vi "Image Processing.vi"(0 "File Path":path, 1 "Lithography Information":T2(array[cluster]), 2 "Crop?":bool, 3 "Crop Data":T3, 4 "Angle (degrees)":dbl, 5 "error in (no error)":errorcluster, 6 "Size":cluster{"Width":dbl, "Height":dbl}, 7 "Page":i32) -> (14 "Image Out":T4(plugin-control), 15 "Offset":T1, 16 "Sample Size":cluster{"Width (µm)":dbl, "Height (µm)":dbl}, 19 "error out":errorcluster)   [LabVIEW 2011]
uses:
  <vilib>/vision/NI_Vision_Development_Module.lvlib
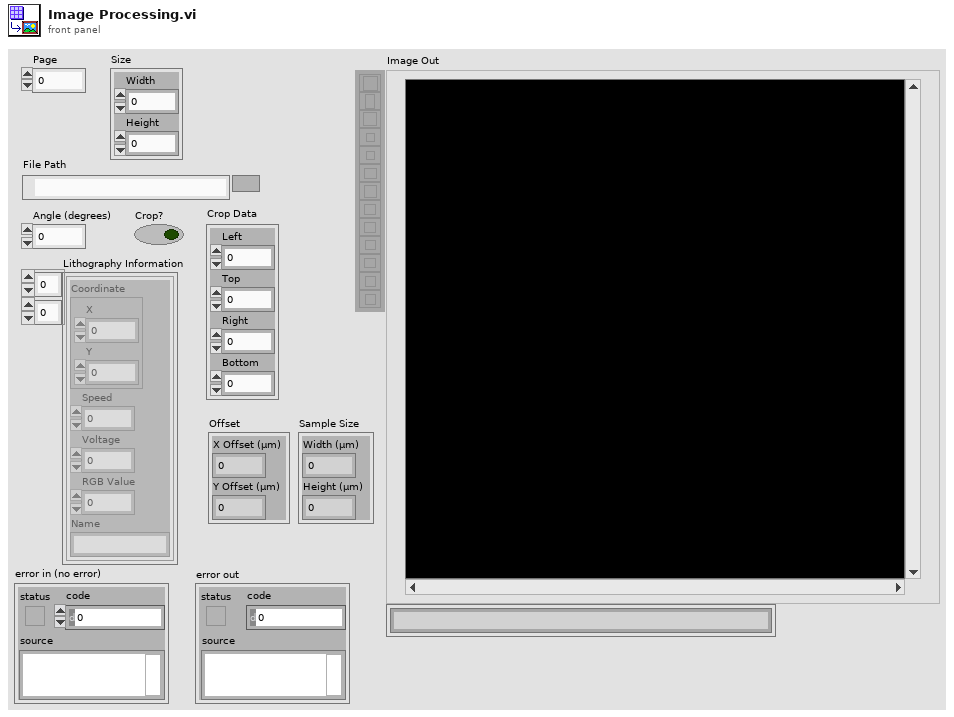
[diagram p1: front panel]
types:
  T1 = cluster{"X Offset (µm)":dbl, "Y Offset (µm)":dbl}
  T2 = cluster{"Coordinate":cluster{"X":dbl, "Y":dbl}, "Speed":dbl, "Voltage":dbl, "RGB Value":i32, "Name":string}[][]
  T3 = cluster{"Left":dbl, "Top":dbl, "Right":dbl, "Bottom":dbl}
  T4 = typedef "IMAQ Image.ctl" = refnum<image>
  T5 = typedef "Image Type" = u32
  T6 = cluster{"Coordinate":cluster{"X":dbl, "Y":dbl}, "Speed":dbl, "Voltage":dbl, "RGB Value":i32, "Name":string}
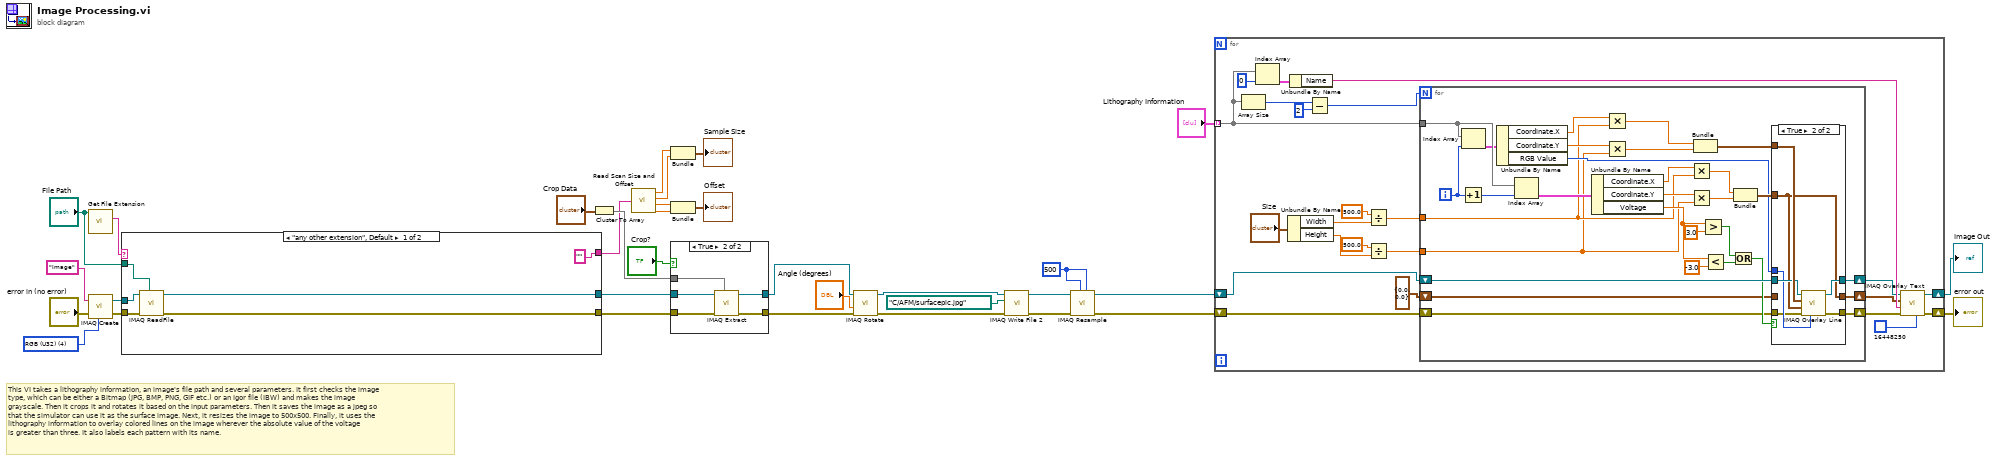
[diagram p0: block diagram]
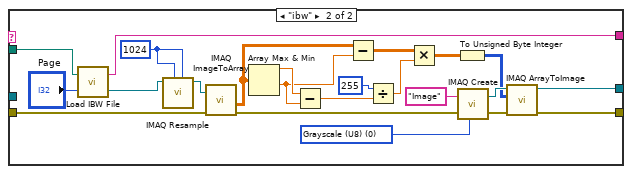
[diagram p2: hidden frame]
diagram:
  w10 = 500 ("Y Resolution")
  w32 = T5 4 items=["Grayscale (U8)", "Grayscale (I16)", "Grayscale (SGL)", "Complex (CSG)", "RGB (U32)", "HSL (U32)", "RGB (U64)", "Grayscale (U16)"] ("Image Type")
  # "This VI takes a lithography information, an image's file path and several parameters. It first checks the image \ntype, which can be either a Bitmap (JPG, BMP, PNG, GIF etc.) or an Igor file (IBW) and makes the image \ngrayscale. Then it crops it and rotates it based on the input parameters. Then it saves the image as a jpeg so \nthat the simulator can use it as the surface image. Next, it resizes the image to 500x500. Finally, it uses the \nlithography information to overlay colored lines on the image wherever the absolute value of the voltage \nis greater than three. It also labels each pattern with its name."
  n1 = call <vilib>:"Get File Extension.vi"("file"="File Path") -> ("lowercase file extension"=w19:string)  [unwired: 7 in, 3 out]
  n2 = call "IMAQ Create"("Image Name"="Image", "Image Type"=w32, "error in (no error)"="error in (no error)") -> ("New Image"=w31:T4, "error out"=w30:errorcluster)  [unwired: 2 in]
  n3 = case shown="\"any other extension\", Default" w19 {
    tunnel: w31 -> [w39 _]
    tunnel: w30 -> [w38 w60]
    tunnel: [w37 w53] -> w29
    tunnel: [w36 w52] -> w28
    tunnel: "File Path" -> [w35 w62]
    tunnel: ["" ("Wave Note") w40] -> w7
    frame "any other extension", Default {
      n4 = call "IMAQ ReadFile"("File Path"=w35, "error in (no error)"=w38, "Image"=w39) -> ("error out"=w36:errorcluster, "Image Out"=w37:T4)  [unwired: 4 in, 3 out]
    }
    frame "ibw" {
      w50 = 1024 ("Y Resolution")
      w57 = T5 0 items=["Grayscale (U8)", "Grayscale (I16)", "Grayscale (SGL)", "Complex (CSG)", "RGB (U32)", "HSL (U32)", "RGB (U64)", "Grayscale (U16)"] ("Image Type")
      n5 = call "Load IBW File.vi"("Page"="Page", "file path (dialog if empty)"=w62) -> ("Image"=w49:T4, "Wave Note"=w40:string)
      n6 = call "IMAQ Resample"("X Resolution"=w50, "Y Resolution"=w50, "Image Src"=w49) -> ("Image Dst Out"=w48:T4)  [unwired: 7 in, 1 out]
      n7 = call "IMAQ ImageToArray"("error in (no error)"=w60, "Image"=w48) -> ("Image Pixels (Float)"=w59:sgl[][], "error out"=w54:errorcluster)  [unwired: 2 in, 3 out]
      n8 = Array Max & Min(array=w59) -> (max value=w47:sgl, min value=w46:sgl)  [unwired: 2 out]
      n9 = Subtract(x=w47, y=w46) -> (x-y=w44:sgl)
      n10 = Subtract(x=w59, y=w46) -> (x-y=w45:sgl[][])
      n11 = Divide(x=255, y=w44) -> (x/y=w42:sgl)
      n12 = Multiply(x=w45, y=w42) -> (x*y=w41:sgl[][])
      n13 = To Unsigned Byte Integer(number=w41) -> (unsigned 8bit integer=w56:u8[][])
      n14 = call "IMAQ Create"("Image Name"="Image", "Image Type"=w57, "error in (no error)"=w54) -> ("New Image"=w58:T4, "error out"=w55:errorcluster)  [unwired: 2 in]
      n15 = call "IMAQ ArrayToImage"("error in (no error)"=w55, "Image Pixels (U8)"=w56, "Image"=w58) -> ("error out"=w52:errorcluster, "Image Out"=w53:T4)  [unwired: 7 in]
    }
  }
  n16 = Cluster To Array(cluster="Crop Data") -> (array=w26:dbl[])
  n17 = call "Read Scan Size and Offset.vi"("Read in the string file"=w7) -> ("X Range (µm)"=w6:dbl, "Y Range (µm)"=w5:dbl, "X Offset (µm)"=w3:dbl, "Y Offset (µm)"=w2:dbl)  [unwired: 4 in]
  n18 = Bundle("X Range (µm)"=w6, "Y Range (µm)"=w5) -> (→"Sample Size":cluster{"X Range (µm)":dbl, "Y Range (µm)":dbl})  [unwired: 1 in]
  n19 = Bundle("X Offset (µm)"=w3, "Y Offset (µm)"=w2) -> (→"Offset":T1)  [unwired: 1 in]
  n20 = case shown="True" "Crop?" {
    tunnel: w29 -> [w64 w68]
    tunnel: w28 -> [w63 w67]
    tunnel: w26 -> [_ w69]
    tunnel: [w64 w65] -> w17
    tunnel: [w63 w66] -> w16
    frame False {
    }
    frame True {
      n21 = call "IMAQ Extract"("Optional Rectangle"=w69, "error in (no error)"=w67, "Image Src"=w68) -> ("error out"=w66:errorcluster, "Image Dst Out"=w65:T4)  [unwired: 7 in]
    }
  }
  n22 = call "IMAQ Rotate"("error in (no error)"=w16, "Angle (degrees)"="Angle (degrees)", "Image Src"=w17) -> ("error out"=w13:errorcluster, "Image Dst Out"=w14:T4)  [unwired: 7 in]
  n23 = call-poly "IMAQ Write File 2"("error in (no error)"=w13, "File Path"=path "C:/AFM/surfacepic.jpg", "Image"=w14) -> ("error out"=w11:errorcluster, "Image Out (duplicate)"=w12:T4)  [unwired: 7 in]
  n24 = call "IMAQ Resample"("X Resolution"=w10, "Y Resolution"=w10, "error in (no error)"=w11, "Image Src"=w12) -> ("error out"=w8:errorcluster, "Image Dst Out"=w9:T4)  [unwired: 6 in]
  n25 = for {
    tunnel: "Lithography Information" -> [w79] mode=indexing
    shift-right: [w81] -> w21
    shift-left: w9 -> [w87]
    shift-right: [w83] -> w24
    shift-left: w8 -> [w89]
    n26 = Array Size(array=w79) -> (size(s)=w92:i32)
    n27 = Index Array(array=w79, index=0) -> (element=w77:T6)
    n28 = Unbundle By Name("Size") -> ("Width"=w71:dbl, "Height"=w70:dbl)
    n29 = Unbundle By Name(w77) -> ("Name"=w86:string)
    n30 = Subtract(x=w92, y=2) -> (x-y=w90:i32)
    n31 = Divide(x=500.0, y=w71) -> (x/y=w74:dbl)
    n32 = Divide(x=500.0, y=w70) -> (x/y=w73:dbl)
    n33 = for {
      N: w90 -> [_]
      tunnel: w79 -> [w100]
      shift-right: [w108] -> w82
      shift-left: w87 -> [w117]
      shift-right: [w101] -> w84
      shift-left: w89 -> [w102]
      tunnel: w74 -> [w96]
      shift-right: [w95] -> w80
      shift-left: cluster{dbl, dbl} {0.0, 0.0} -> [w94]
      tunnel: w73 -> [w93]
      i -> [w99]
      n34 = Increment(x=w99) -> (x+1=w118:i32)
      n35 = Index Array(array=w100, index=w99) -> (element=w98:T6)
      n36 = Unbundle By Name(w98) -> ("Coordinate.X"=w122:dbl, "Coordinate.Y"=w121:dbl, "RGB Value"=w109:i32)
      n37 = Index Array(array=w100, index=w118) -> (element=w115:T6)
      n38 = Unbundle By Name(w115) -> ("Coordinate.X"=w113:dbl, "Coordinate.Y"=w114:dbl, "Voltage"=w97:dbl)
      n39 = Multiply(x=w122, y=w96) -> (x*y=w120:dbl)
      n40 = Multiply(x=w121, y=w93) -> (x*y=w119:dbl)
      n41 = Multiply(x=w113, y=w96) -> (x*y=w112:dbl)
      n42 = Multiply(x=w114, y=w93) -> (x*y=w111:dbl)
      n43 = Bundle(w120, w119) -> (w116:cluster{dbl, dbl})  [unwired: 1 in]
      n44 = Greater?(x=w97, y=3.0) -> (0:w105:bool)
      n45 = Less?(x=w97, y=-3.0) -> (x < y?=w104:bool)
      n46 = Or(x=w105, y=w104) -> (x .or. y?=w103:bool)
      n47 = Bundle(w112, w111) -> (w110:cluster{dbl, dbl})  [unwired: 1 in]
      n48 = case shown="True" w103 {
        tunnel: w117 -> [w125 w130]
        tunnel: w116 -> [_ w132]
        tunnel: w110 -> [_ w126]
        tunnel: w109 -> [_ w129]
        tunnel: [w125 w131] -> w108
        tunnel: w102 -> [w124 w128]
        tunnel: [w124 w127] -> w101
        tunnel: [w123 w126] -> w95
        tunnel: w94 -> [w123 _]
        frame False {
        }
        frame True {
          n49 = call "IMAQ Overlay Line"("Color"=w129, "error in (no error)"=w128, "End Point"=w126, "Start Point"=w132, "Image"=w130) -> ("error out"=w127:errorcluster, "Image Out"=w131:T4)  [unwired: 5 in]
        }
      }
    }
    n50 = call "IMAQ Overlay Text"("BG Color (Transparent)"=u32 16448250, "error in (no error)"=w84, "String"=w86, "Origin"=w80, "Image"=w82) -> ("error out"=w83:errorcluster, "Image Out"=w81:T4)  [unwired: 5 in]
  }
  "Image Out" <- w21
  "error out" <- w24
